vi "Test Connection Callback.vi"(7 "Owner":refnum<class>, 8 "error in (no error)":errorcluster, 10 "Connection State":T1, 11 "Connection":refnum<class "Connection.lvclass">) -> (0 "error out":errorcluster)   [LabVIEW 2020]
uses:
  <vilib>/IlluminatedG/lv-stream/Connection/Connection.lvclass
  <vilib>/IlluminatedG/lv-stream/Connection State.ctl
  Stream-Websocket/WebsocketStream/WebsocketStream.lvclass
  <vilib>/IlluminatedG/lv-stream/Stream.lvlib
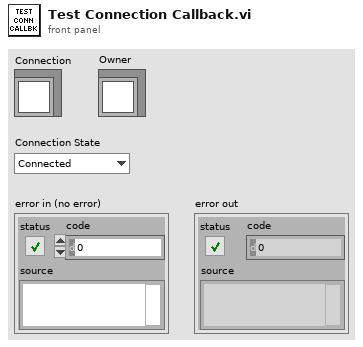
[diagram p1: front panel]
types:
  T1 = typedef "Stream.lvlib/Connection State.ctl" = enum16{"Connected", "Disconnected"}
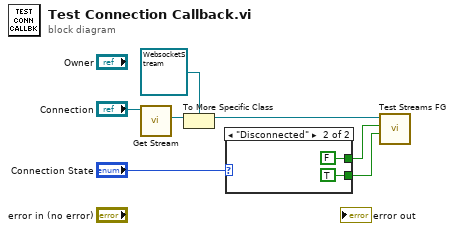
[diagram p0: block diagram]
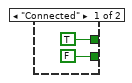
[diagram p2: hidden frame]
diagram:
  n1 = call-dynamic "Get Stream.vi"("Connection in"="Connection") -> ("Stream"=w6:refnum<class "Stream.lvclass">)  [unwired: 8 in, 2 out]
  n2 = To More Specific Class(target class=refnum<class "WebsocketStream.lvclass"> refnum ("Stream-Websocket.lvlib:WebsocketStream.lvclass"), reference=w6) -> (specific class reference=w2:refnum<class "WebsocketStream.lvclass">)  [unwired: 1 in, 1 out]
  n3 = case shown="\"Disconnected\"" "Connection State" {
    tunnel: [TRUE ("Add") FALSE ("Add")] -> w3
    tunnel: [FALSE ("Add") TRUE ("Add")] -> w1
    frame "Connected" {
    }
    frame "Disconnected" {
    }
  }
  n4 = call "Test Streams FG.vi"("Remove"=w1, "Add"=w3, "Stream"=w2) -> ()  [unwired: 8 in, 1 out]
